vi "WaitForServerStartup.vi"(0 "ROS in":T2={"topic port"=0, "Node"="", "topic"="", "type"="", "node port"=0, "error "={"status"=FALSE, "code"=0, "source"=""}, "Direction"=enum."Node", "APIs"=[], "Update (ms)"=1, "write queue"=1}) -> (1 "success?":bool, 2 "ROS out":T2={"topic port"=0, "Node"="", "topic"="", "type"="", "node port"=0, "error "={"status"=FALSE, "code"=0, "source"=""}, "Direction"=enum."Node", "APIs"=[], "Update (ms)"=1, "write queue"=1})   [LabVIEW 2010]
uses:
  <userlib>/ROSforLV/ROS/Code/SubVIs/_ROSControl.ctl
  <userlib>/ROSforLV/ROS/Code/SubVIs/_ROSDirection.ctl
  <userlib>/ROSforLV/ROS/Code/Console/Servers/ServerSubs/MyState.ctl
panel:
  out "data":T1
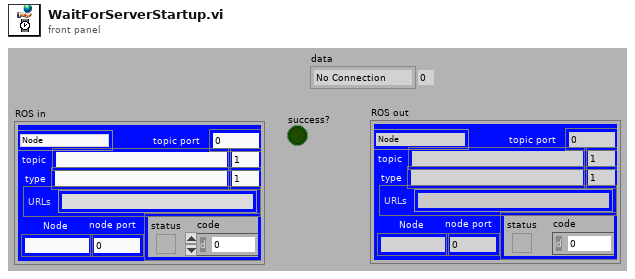
[diagram p1: front panel]
types:
  T1 = typedef "MyState.ctl" = enum16{"No Connection", "Registered", "Connected", "Close"}
  T2 = typedef "_ROSControl.ctl" = cluster{"topic port":u16, "Node":string, "topic":string, "type":string, "node port":u32, "error ":errorcluster, "Direction":T3, "APIs":string[], "Update (ms)":u16, "write queue":u16}
  T3 = typedef "_ROSDirection.ctl" = enum16{"Node", "Publisher", "Subscriber", "Service Client"}
  T4 = typedef "ServoInfo.ctl" = cluster{"vi name":string, "VI Refnum":refnum<vi>, "queue":refnum<queue>, "ROS":T2, "notifier":refnum<notifier>}
  T5 = enum32{"Bad", "Idle", "Run top level", "Running"}
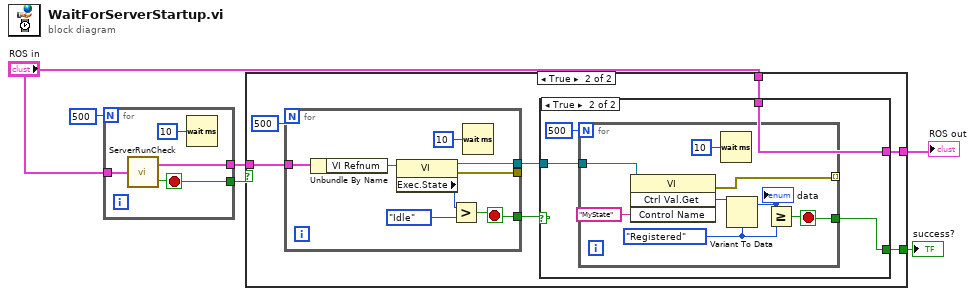
[diagram p0: block diagram]
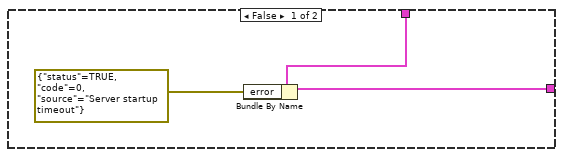
[diagram p2: hidden frame]
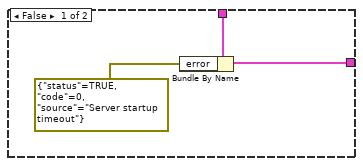
[diagram p3: hidden frame]
diagram:
  n1 = for {
    N: 500 -> [_]
    tunnel: "ROS in" -> [w10]
    tunnel: [w8] -> w5
    tunnel: [w7] -> w4
    stop <- w8 stop-if-true
    n2 = call <userlib>:"ServerRunCheck.vi"("ROS in"=w10) -> ("Running?"=w8:bool, "ServerFound"=w7:T4)
    n3 = Wait (ms)(milliseconds to wait=u32 10) -> ()  [unwired: 1 out]
  }
  n4 = case shown="True" w5 {
    tunnel: w4 -> [_ w20]
    tunnel: [_ w17] -> w3
    tunnel: [w12 w16] -> w1
    tunnel: "ROS in" -> [w13 w15]
    frame False {
      n5 = Bundle By Name(cluster=w13, "error"=errorcluster {"status"=TRUE, "code"=0, "source"="Server startup timeout"}) -> (w12:T2)
    }
    frame True {
      n6 = for {
        N: 500 -> [_]
        tunnel: w20 -> [w40]
        tunnel: [w39] -> _
        tunnel: [w38] -> w18
        tunnel: [w36] -> w14
        stop <- w38 stop-if-true
        n7 = Unbundle By Name(w40) -> ("VI Refnum"=w43:refnum<vi>)
        n8 = property class="VI"(reference=w43) -> (reference out=w36:refnum<vi>, error out=w39:errorcluster, "Exec.State"=w41:T5)  [unwired: 1 in]
        n9 = Greater?(x=w41, y=T5."Idle" ("Execution:State")) -> (0:w38:bool)
        n10 = Wait (ms)(milliseconds to wait=u32 10) -> ()  [unwired: 1 out]
      }
      n11 = case shown="True" w18 {
        tunnel: [_ w24] -> w17
        tunnel: [w22 w27] -> w16
        tunnel: w15 -> [w23 w27]
        tunnel: w14 -> [_ w26]
        frame False {
          n12 = Bundle By Name(cluster=w23, "error"=errorcluster {"status"=TRUE, "code"=0, "source"="Server startup timeout"}) -> (w22:T2)
        }
        frame True {
          n13 = for {
            N: 500 -> [_]
            tunnel: w26 -> [w34]
            tunnel: [w29] -> w24
            tunnel: [w28] -> _ mode=indexing
            stop <- w29 stop-if-true
            w30 = MyState."Registered" ("MyState")
            n14 = invoke class="VI" method="Ctrl Val.Get"(reference=w34, "Control Name"="MyState") -> (error out=w28:errorcluster, "Get Control Value Variant"=w33:variant)  [unwired: 2 in, 2 out]
            n15 = Wait (ms)(milliseconds to wait=u32 10) -> ()  [unwired: 1 out]
            n16 = Variant To Data(Variant=w33, type=w30) -> (data=w31:T1)  [unwired: 1 in, 1 out]
            "data" <- w31
            n17 = Greater Or Equal?(x=w31, y=w30) -> (x >= y?=w29:bool)
          }
        }
      }
    }
  }
  "success?" <- w3
  "ROS out" <- w1
